vi "Panel.vi"(11 "DA Parent in":refnum<class "DA Parent.lvclass">) -> ()   [LabVIEW 2014, in "Display As.lvlib" / "DA Parent.lvclass"]
uses:
  DA Parent.lvclass
  OOPanel/Panel/Panel.lvclass
panel:
  out "Value":string
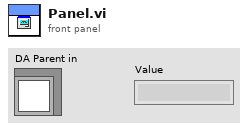
[diagram p1: front panel]
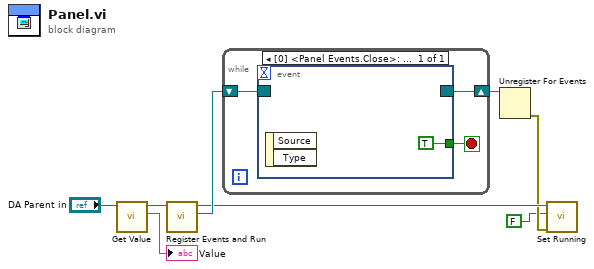
[diagram p0: block diagram]
diagram:
  n1 = call-dynamic "Get Value.vi"("DA Parent in"="DA Parent in") -> ("Value"=→"Value":string, "DA Parent out"=w6:refnum<class "DA Parent.lvclass">)  [unwired: 8 in, 1 out]
  n2 = call "Register Events and Run.vi"("Panel in"=w6) -> ("Panel Event Reg"=w5:refnum<event-registration>, "Panel out"=w3:refnum<class "DA Parent.lvclass">)  [unwired: 8 in, 1 out]
  n3 = while {
    shift-right: [w10] -> w4
    shift-left: w5 -> [w11]
    stop <- w9 stop-if-true
    n4 = event shown="[0] <Panel Events.Close>: User Event" {
      selector: w11 -> [_]
      dyn-events: [_] -> w10
      timeout: _ -> [_]
      tunnel: [TRUE] -> w9
      event User Event {
        n5 = event-data() -> ()  [unwired: 1 in, 2 out]
      }
    }
  }
  n6 = Unregister For Events(event registration refnum=w4) -> (error out=w2:errorcluster)  [unwired: 1 in]
  n7 = call "Set Running.vi"("error in (no error)"=w2, "Running"=FALSE, "Panel in"=w3) -> ()  [unwired: 7 in, 2 out]
